vi "read.vi"(8 "error in (no error)":errorcluster, 10 "Name":string, 11 "BaseSetting in":refnum<class "Setting.lvclass">) -> (0 "error out":errorcluster, 1 "SettingFilePath":path, 2 "XML":string, 3 "BaseSetting out":refnum<class "Setting.lvclass">)   [LabVIEW 2016, in "Settings.lvlib" / "Setting.lvclass"]
uses:
  Setting.lvclass
  Setting.lvclass/Setting.ctl
  <vilib>/Utility/xml.llb/Read From XML File(string).vi
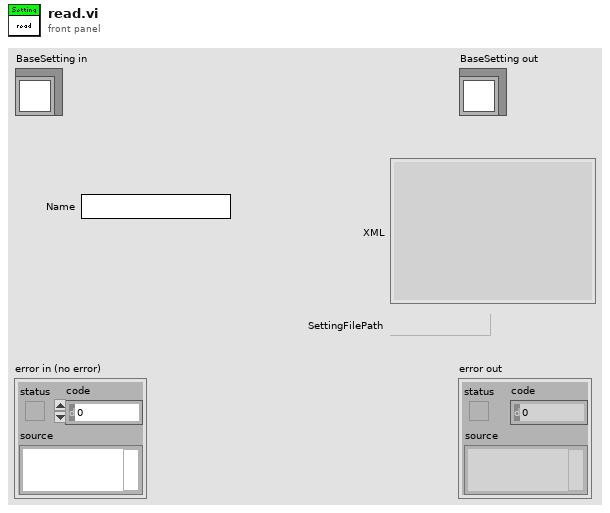
[diagram p1: front panel]
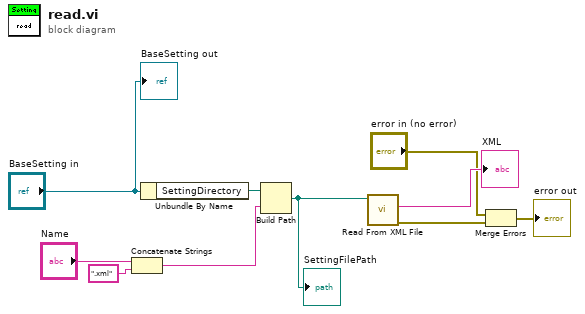
[diagram p0: block diagram]
diagram:
  n1 = Concatenate Strings("Name", ".xml") -> (w8:string)
  n2 = Unbundle By Name("BaseSetting in") -> ("SettingDirectory"=w7:path)
  n3 = Build Path(base path=w7, name or relative path=w8) -> (appended path=w10:path)
  "SettingFilePath" <- w10
  n4 = call-poly <vilib>:"Read From XML File.vi"("XML File Path"=w10) -> ("error out"=w4:errorcluster, "XML Elements"=→"XML":string)  [unwired: 8 in, 1 out]
  n5 = Merge Errors("error in (no error)", w4) -> (→"error out":errorcluster)
  "BaseSetting out" <- "BaseSetting in"
